vi "Config Sound Card.vi"(3 "error in":errorcluster, 4 "Samples Per Read":i32, 5 "Song":path) -> (0 "error out":errorcluster, 1 "task ID":T1 format="%.0x", 2 "sound file refnum":T2)   [LabVIEW 2011, in "LabVIEW Interface for Arduino.lvlib"]
uses:
  <vilib>/sound2/lvsound2.llb/Sound File Refnum.ctl
  <vilib>/sound2/lvsound2.llb/Sound Output Task ID.ctl
  <vilib>/sound2/lvsound2.llb/Sampling Mode.ctl
  <vilib>/sound2/lvsound2.llb/Sound File Info (path).vi
  <vilib>/sound2/lvsound2.llb/Sound File Read Open.vi
  <vilib>/LabVIEW Interface for Arduino/LabVIEW Interface for Arduino.lvlib
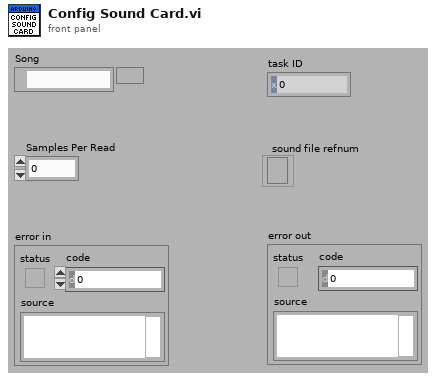
[diagram p1: front panel]
types:
  T1 = typedef "Sound Output Task ID.ctl" = u32
  T2 = typedef "Sound File Refnum.ctl" = refnum<file>
  T3 = typedef "Sampling Mode.ctl" = i32
  T4 = typedef "Sound Data Format.ctl" = cluster{"sample rate (S/s)":dbl, "number of channels":i32, "bits per sample":i32}
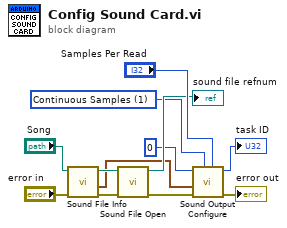
[diagram p0: block diagram]
diagram:
  w3 = T3 1 items=["Finite Samples", "Continuous Samples"] ("sample mode")
  n1 = call-poly <vilib>:"Sound File Info.vi"("error in (no error)"="error in", "path"="Song") -> ("error out"=w6:errorcluster, "sound format"=w2:T4, "path out"=w9:path)  [unwired: 6 in, 1 out]
  n2 = call-poly <vilib>:"Sound File Open.vi"("error in (no error)"=w6, "path"=w9) -> ("error out"=w7:errorcluster, "sound file refnum"=→"sound file refnum":T2)  [unwired: 8 in]
  n3 = call <vilib>:"Sound Output Configure.vi"("number of samples/ch"="Samples Per Read", "sample mode"=w3, "error in (no error)"=w7, "sound format"=w2, "device ID"=u32 0) -> ("error out"=→"error out":errorcluster, "task ID"=→"task ID":T1)  [unwired: 5 in]
